vi "myRIO_BRig_RT_dataTrial_LR_Reward_Event_l2.vi"() -> (2 "output_LR_Reward_Event_l2":i32)   [LabVIEW 2014]
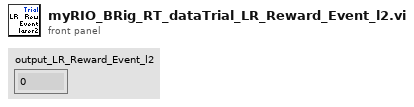
[diagram p1: front panel]
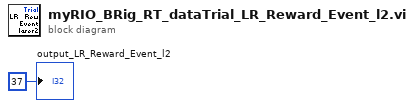
[diagram p0: block diagram]
diagram:
  "output_LR_Reward_Event_l2" <- 37 ("output_iBlock")
